vi "Waveforms Generation Main Page.vi"(8 "error in (no error)":errorcluster, 11 "Node Ptr":T1 format="%.0x") -> (0 "error out":errorcluster)   [LabVIEW 2013, in "Waveforms Generation Custom Device.lvlib"]
uses:
  Waveforms Generation Custom Device.lvlib
  <vilib>/NI Veristand/Custom Device API/Custom Device Item Ref.ctl
  <vilib>/NI Veristand/Custom Device API/Get Item Property (Double).vi
  <vilib>/NI Veristand/Custom Device API/Set Item Property (Double).vi
  <vilib>/NI Veristand/Custom Device API/Custom Device API.lvlib
panel:
  out "Version":string
  in  "Number of Samples per Waveform":dbl=10.0 min=10.0 max=1000000.0 step=1.0 format="%#_6p"
  in  "dt":dbl=1e-07 min=1e-07 max=0.1 step=0.001 format="%#_6p"
  in  "Header":cluster{"Section Name":string}={"Section Name"="Waveform Analysis and Generation Settings"}
  out "Description":string
  in  "Name":string
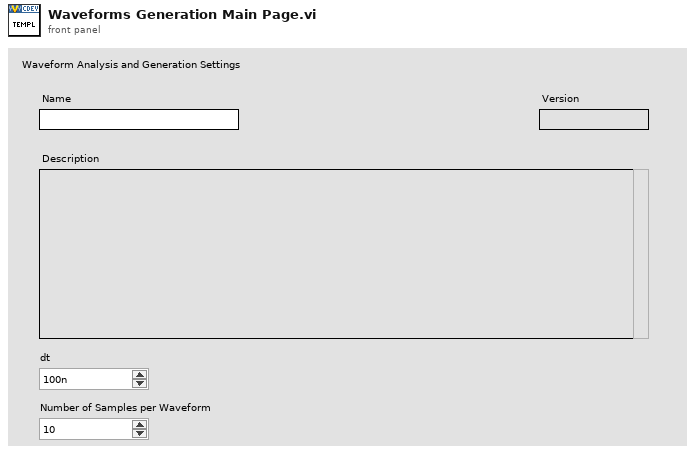
[diagram p1: front panel]
types:
  T1 = typedef "Custom Device API.lvlib/Custom Device Item Ref.ctl" = u64
  T2 = typedef "Custom Device API.lvlib/Custom Device Item Info.ctl" = cluster{"Name":string, "Is Channel":bool, "GUID":string, "Is Waveform":bool}
  T3 = typedef "Custom Device API.lvlib/Custom Device Commands.ctl" = enum16{"Default", "Item renamed", "Shutdown", "Dynamic button pressed"}
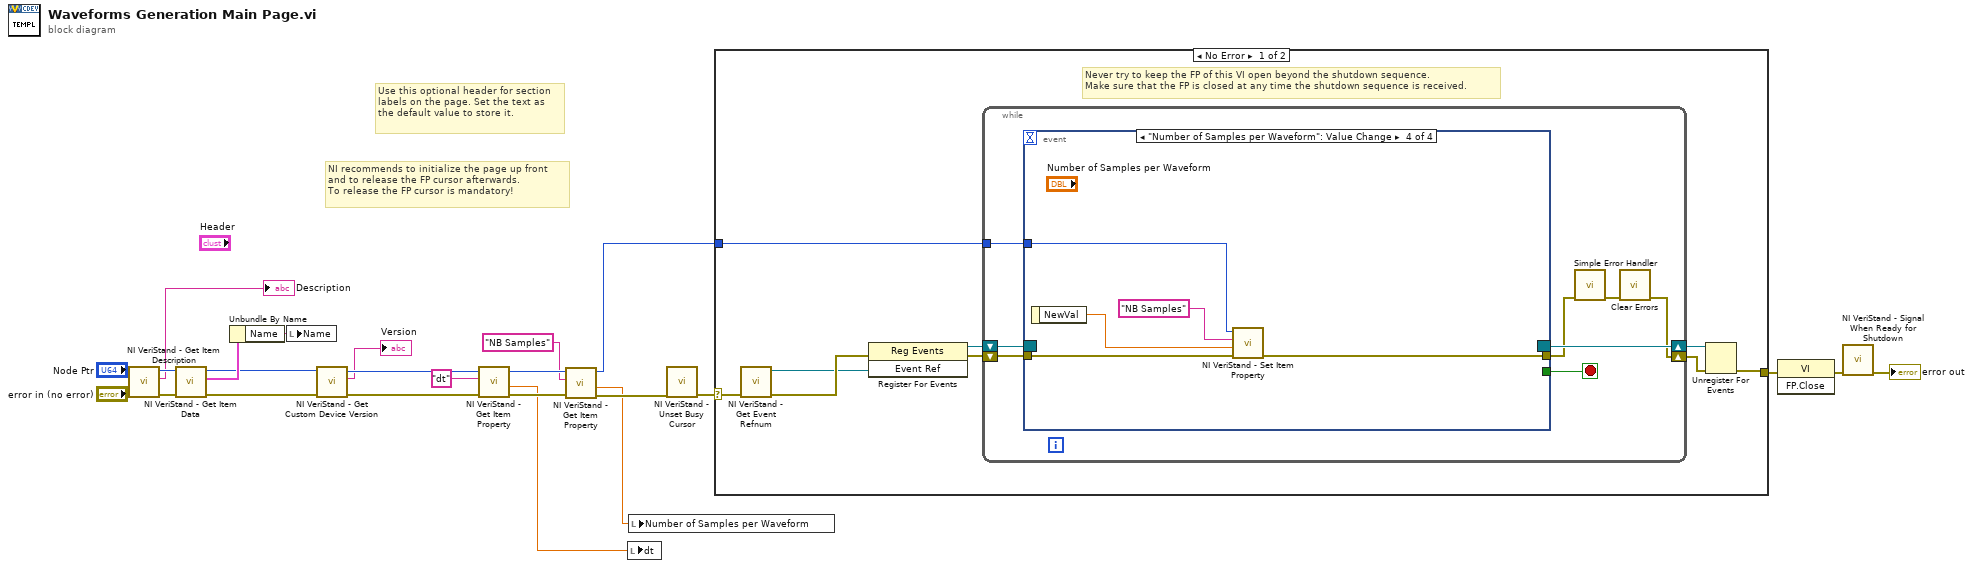
[diagram p0: block diagram]
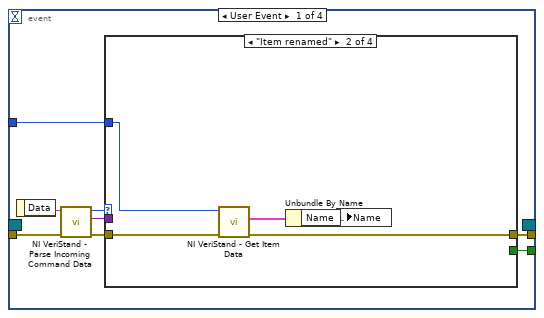
[diagram p2: hidden frame]
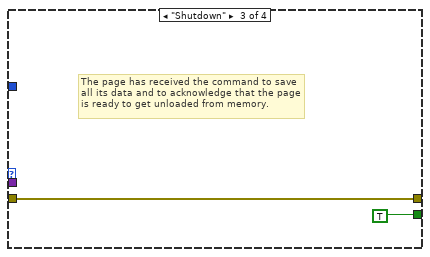
[diagram p4: hidden frame]
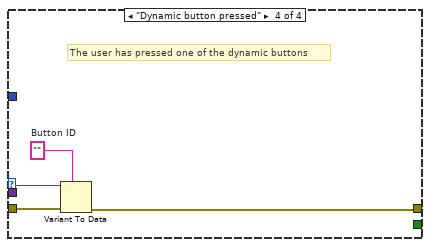
[diagram p5: hidden frame]
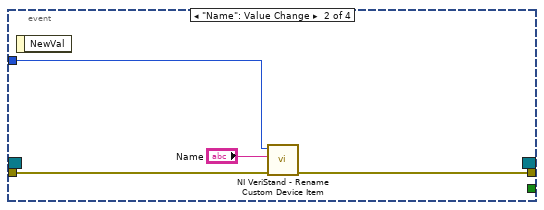
[diagram p6: hidden frame]
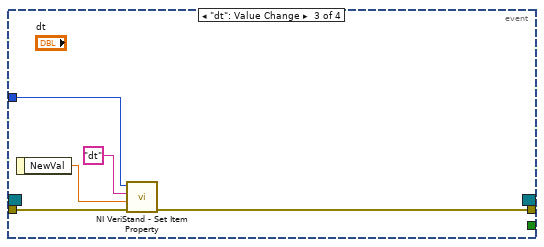
[diagram p7: hidden frame]
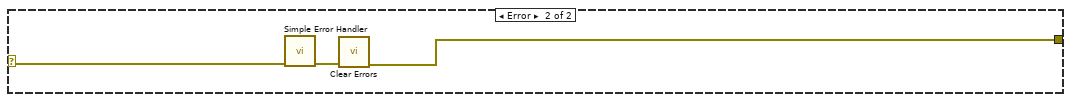
[diagram p8: hidden frame]
diagram:
  # "Use this optional header for section labels on the page. Set the text as the default value to store it."
  # "NI recommends to initialize the page up front\nand to release the FP cursor afterwards.\nTo release the FP cursor is mandatory!"
  n1 = call <vilib>:"NI VeriStand - Get Item Description.vi"("error in (no error)"="error in (no error)", "Item Ref in"="Node Ptr") -> ("error out"=w19:errorcluster, "Description"=→"Description":string, "Item Ref out"=w20:T1)  [unwired: 7 out]
  n2 = call <vilib>:"NI VeriStand - Get Item Data.vi"("error in (no error)"=w19, "Item Ref in"=w20) -> ("error out"=w4:errorcluster, "Item Info"=w18:T2, "Item Ref out"=w5:T1)  [unwired: 7 out]
  n3 = Unbundle By Name(w18) -> ("Name"=w17:string)
  n4 = local write "Name"(w17) -> ()
  n5 = call <vilib>:"NI VeriStand - Get Custom Device Version.vi"("error in (no error)"=w4, "Device Ref in"=w5) -> ("error out"=w3:errorcluster, "Value"=→"Version":string, "Device Ref out"=w2:T1)  [unwired: 7 in]
  n6 = call-poly <vilib>:"NI VeriStand - Get Item Property.vi"("error in (no error)"=w3, "Property Name"="dt", "Item Ref in"=w2) -> ("error out"=w12:errorcluster, "Value"=w6:dbl, "Item Ref out"=w10:T1)  [unwired: 5 in, 1 out]
  n7 = call-poly <vilib>:"NI VeriStand - Get Item Property.vi"("error in (no error)"=w12, "Property Name"="NB Samples", "Item Ref in"=w10) -> ("error out"=w11:errorcluster, "Value"=w7:dbl, "Item Ref out"=w9:T1)  [unwired: 5 in, 1 out]
  n8 = local write "dt"(w6) -> ()
  n9 = local write "Number of Samples per Waveform"(w7) -> ()
  n10 = call <vilib>:"NI VeriStand - Unset Busy Cursor.vi"("error in (no error)"=w11) -> ("error out"=w21:errorcluster)  [unwired: 10 out]
  n11 = case shown="No Error" w21 {
    selector: w21 -> [w27 w78]
    tunnel: [w26 w76] -> w24
    tunnel: w9 -> [w25 _]
    frame No Error {
      # "Never try to keep the FP of this VI open beyond the shutdown sequence.\nMake sure that the FP is closed at any time the shutdown sequence is received."
      n12 = call <vilib>:"NI VeriStand - Get Event Refnum.vi"("error in (no error)"=w27) -> ("error out"=w33:errorcluster, "Event Ref"=w30:refnum<user-event>)  [unwired: 9 out]
      n13 = register-events(error in=w33, w30) -> (reference out=w28:refnum<event-registration>, error out=w29:errorcluster)  [unwired: 1 in]
      n14 = while {
        shift-right: [w35] -> w31
        shift-left: w29 -> [w40]
        shift-right: [w41] -> w32
        shift-left: w28 -> [w39]
        tunnel: w25 -> [w34]
        stop <- w38 stop-if-true
        n15 = event shown="[3] \"Number of Samples per Waveform\": Value Change" {
          selector: w39 -> [_ _ _ _]
          dyn-events: [_ _ _ _] -> w41
          timeout: _ -> [_ _ _ _]
          tunnel: w40 -> [w49 w65 w69 w73]
          tunnel: [w45 _ _ _] -> w38
          tunnel: [w44 w64 w67 w71] -> w37
          tunnel: w34 -> [w42 w62 w66 w74]
          event User Event {
            n16 = event-data() -> ("Data"=w48:string)  [unwired: 1 out]
            n17 = call <vilib>:"NI VeriStand - Parse Incoming Command Data.vi"("error in (no error)"=w49, "Incoming data"=w48) -> ("error out"=w47:errorcluster, "Outgoing data"=w43:variant, "Action"=w46:T3)  [unwired: 7 out]
            n18 = case shown="\"Item renamed\"" w46 {
              tunnel: w47 -> [w50 w55 w56 w61]
              tunnel: [_ _ TRUE _] -> w45
              tunnel: [w50 w53 w56 w58] -> w44
              tunnel: w43 -> [_ _ _ w60]
              tunnel: w42 -> [_ w51 _ _]
              frame "Default", Default {
              }
              frame "Item renamed" {
                n19 = call <vilib>:"NI VeriStand - Get Item Data.vi"("error in (no error)"=w55, "Item Ref in"=w51) -> ("error out"=w53:errorcluster, "Item Info"=w54:T2)  [unwired: 8 out]
                n20 = Unbundle By Name(w54) -> ("Name"=w52:string)
                n21 = local write "Name"(w52) -> ()
              }
              frame "Shutdown" {
                # "The page has received the command to save all its data and to acknowledge that the page is ready to get unloaded from memory."
              }
              frame "Dynamic button pressed" {
                w59 = ""  # Button ID
                # "The user has pressed one of the dynamic buttons"
                n22 = Variant To Data(error in=w61, type=w59, Variant=w60) -> (error out=w58:errorcluster)  [unwired: 1 out]
              }
            }
          }
          event "Name": Value Change {
            n23 = event-data() -> ()  [unwired: 2 out]
            n24 = call <vilib>:"NI VeriStand - Rename Custom Device Item.vi"("error in (no error)"=w65, "New Name"="Name", "Item Ref in"=w62) -> ("error out"=w64:errorcluster)  [unwired: 1 in, 7 out]
          }
          event "dt": Value Change {
            n25 = event-data() -> ("NewVal"=w68:dbl)  [unwired: 1 out]
            n26 = call-poly <vilib>:"NI VeriStand - Set Item Property.vi"("error in (no error)"=w69, "Value"=w68, "Property Name"="dt", "Item Ref in"=w66) -> ("error out"=w67:errorcluster)  [unwired: 5 in, 2 out]
          }
          event "Number of Samples per Waveform": Value Change {
            n27 = event-data() -> ("NewVal"=w72:dbl)  [unwired: 1 out]
            n28 = call-poly <vilib>:"NI VeriStand - Set Item Property.vi"("error in (no error)"=w73, "Value"=w72, "Property Name"="NB Samples", "Item Ref in"=w74) -> ("error out"=w71:errorcluster)  [unwired: 5 in, 2 out]
          }
        }
        n29 = call <vilib>:"Simple Error Handler.vi"("error in (no error)"=w37) -> ("error out"=w36:errorcluster)  [unwired: 1 in, 7 out]
        n30 = call <vilib>:"Clear Errors.vi"("error in (no error)"=w36) -> ("error out"=w35:errorcluster)  [unwired: 6 out]
      }
      n31 = Unregister For Events(event registration refnum=w32, error in=w31) -> (error out=w26:errorcluster)
    }
    frame Error {
      n32 = call <vilib>:"Simple Error Handler.vi"("error in (no error)"=w78) -> ("error out"=w77:errorcluster)  [unwired: 1 in, 7 out]
      n33 = call <vilib>:"Clear Errors.vi"("error in (no error)"=w77) -> ("error out"=w76:errorcluster)  [unwired: 6 out]
    }
  }
  n34 = invoke class="VI" method="FP.Close"(error in=w24) -> (error out=w23:errorcluster)  [unwired: 2 in, 2 out]
  n35 = call <vilib>:"NI VeriStand - Signal When Ready for Shutdown.vi"("error in (no error)"=w23) -> ("error out"=→"error out":errorcluster)  [unwired: 10 out]
